vi "append log_array.vi"(8 "error in (no error)":errorcluster caption="에러 입력(에러 없음)", 10 "log to append":string[](array[string]), 11 "GUI Log Class 입력":refnum<class "GUI Log Class.lvclass">) -> (0 "error out":errorcluster caption="에러 출력", 3 "GUI Log Class 출력":refnum<class "GUI Log Class.lvclass">)   [LabVIEW 2020, in "GUI Log Class.lvclass"]
uses:
  GUI Log Class.lvclass
  GUI Log Class.lvclass/GUI Log Class.ctl
  Accessors/Read appender queue.vi
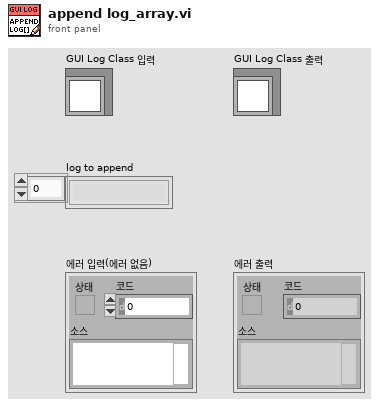
[diagram p1: front panel]
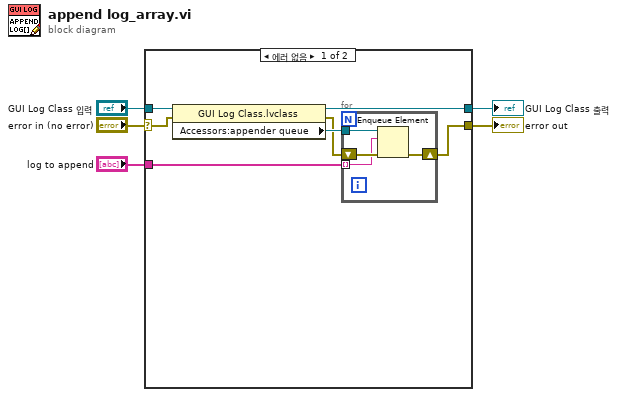
[diagram p0: block diagram]
diagram:
  n1 = case shown="에러 없음" "error in (no error)" {
    selector: "error in (no error)" -> [w9 w18]
    tunnel: [w7 w18] -> w4
    tunnel: [w11 w17] -> w2
    tunnel: "GUI Log Class 입력" -> [w12 w17]
    tunnel: "log to append" -> [w6 _]
    frame No Error {
      n2 = property class="GUI Log Class.lvclass"(reference=w12, error in=w9) -> (reference out=w11:refnum<class "GUI Log Class.lvclass">, error out=w8:errorcluster, "Accessors:appender queue"=w10:refnum<queue>)
      n3 = for {
        tunnel: w10 -> [w16]
        tunnel: w6 -> [w13] mode=indexing
        shift-right: [w14] -> w7
        shift-left: w8 -> [w15]
        n4 = Enqueue Element(queue=w16, element=w13, error in (no error)=w15) -> (error out=w14:errorcluster)  [unwired: 1 in, 2 out]
      }
    }
    frame Error {
    }
  }
  "error out" <- w4
  "GUI Log Class 출력" <- w2
